vi "FileRetrieve.vi"(8 "error in (no error)":errorcluster, 9 "(Empty=No Action)":path caption="To Folder", 10 "(Empty=No Action)":string caption="File Name", 11 "controller in":refnum<k24>) -> (0 "error out":errorcluster, 3 "controller out":refnum<k24>)   [LabVIEW 2010]
uses:
  c:/aerotech/controller/5.xx.xxx/ensemble/pc/labview/2010/bin/Aerotech.Ensemble.dll
  bin/Aerotech.Ensemble.dll
  c:/aerotech/controller/5.xx.xxx/ensemble/pc/labview/2010/bin/Aerotech.Ensemble.LabVIEW.dll
  bin/Aerotech.Ensemble.LabVIEW.dll
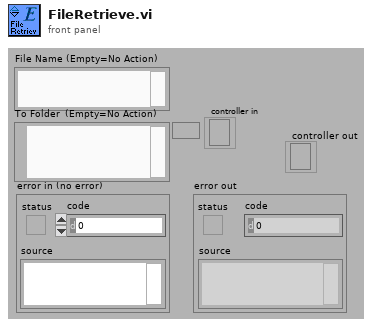
[diagram p1: front panel]
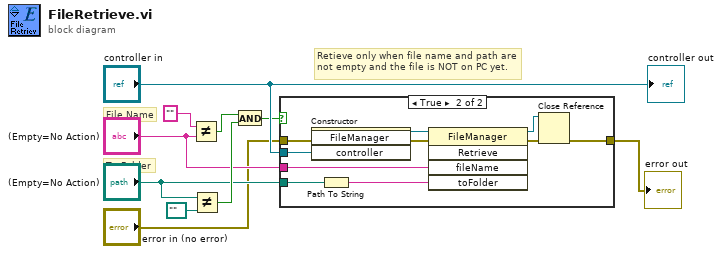
[diagram p0: block diagram]
diagram:
  # "To Folder"
  # "File Name"
  # "Retieve only when file name and path are not empty and the file is NOT on PC yet."
  n1 = Not Equal?(x="", y="(Empty=No Action)") -> (x != y?=w6:bool)
  n2 = Not Equal?(x="(Empty=No Action)", y=path "") -> (x != y?=w5:bool)
  n3 = And(x=w6, y=w5) -> (x .and. y?=w1:bool)
  n4 = case shown="True" w1 {
    tunnel: [w11 w14] -> w10
    tunnel: "(Empty=No Action)" -> [_ w13]
    tunnel: "error in (no error)" -> [w11 w17]
    tunnel: "controller in" -> [_ w16]
    tunnel: "(Empty=No Action)" -> [_ w12]
    frame False {
    }
    frame True {
      n5 = constructor class="FileManager"(error in=w17, "controller"=w16) -> (reference out=w19:refnum<k24>, error out=w18:errorcluster)  [unwired: 2 in, 2 out]
      n6 = Path To String(path=w13) -> (string=w15:string)
      n7 = invoke class="FileManager" method="Retrieve"(reference=w19, error in=w18, "fileName"=w12, "toFolder"=w15) -> (reference out=w20:refnum<k24>, error out=w21:errorcluster)  [unwired: 1 in, 3 out]
      n8 = Close Reference(reference=w20, error in (no error)=w21) -> (error out=w14:errorcluster)
    }
  }
  "error out" <- w10
  "controller out" <- "controller in"
